vi "test 9401 DIO FPGA Mode Loop Back.vi"(8 "error in (no error)":errorcluster, 11 "TestCase in":refnum<class "Scan Engine EtherCAT System Tests.lvclass">) -> (0 "error out":errorcluster, 3 "TestCase out":refnum<class "Scan Engine EtherCAT System Tests.lvclass">)   [LabVIEW 2019, in "Scan Engine EtherCAT System Tests.lvclass"]
uses:
  Scan Engine EtherCAT System Tests.lvclass
  C:/Users/nitest/Desktop/Git 2019/niveristand-custom-device-testing-tools/VeriStandTestCase/VeriStandTestCase.lvclass
  <vilib>/addons/_JKI Toolkits/VI Tester/TestCase.llb/TestCase.lvclass
  niveristand-custom-device-testing-tools/VeriStandTestCase/VeriStandTestCase.lvclass
  C:/Program Files (x86)/National Instruments/LabVIEW 2019/vi.lib/addons/_JKI Toolkits/VI Tester/TestCase.llb/TestCase.lvclass
  Scan Engine Custom Device.lvlib
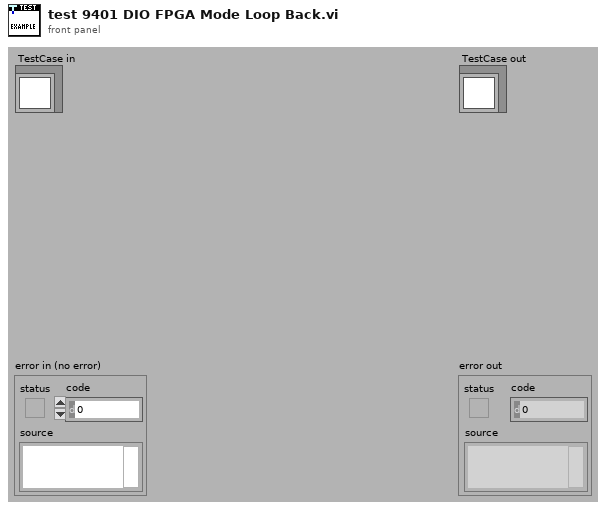
[diagram p1: front panel]
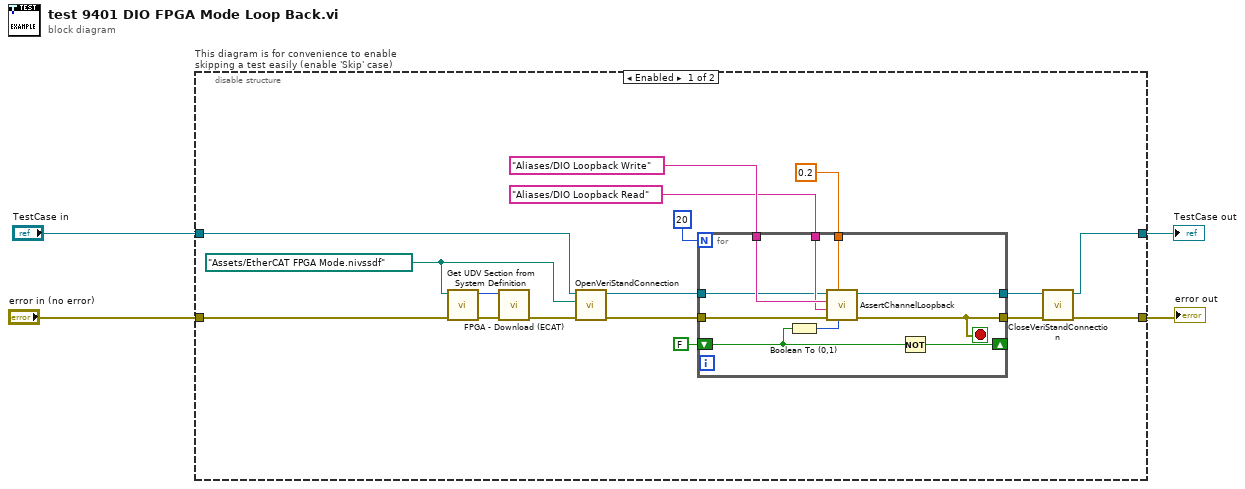
[diagram p0: block diagram]
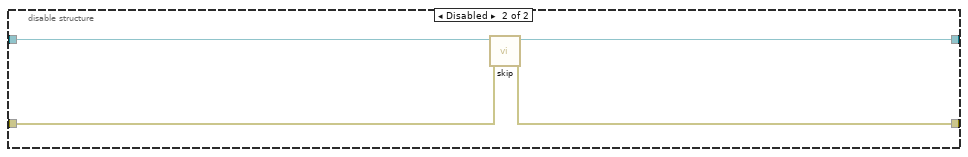
[diagram p2: hidden frame]
diagram:
  n1 = disable-structure "This diagram is for convenience to enable skipping a test easily (enable 'Skip' case)" shown="Enabled" {
    disable-tunnel: "TestCase in" -> [w12 w35]
    disable-tunnel: [w11 w33] -> w1
    disable-tunnel: [w13 w34] -> w3
    disable-tunnel: "error in (no error)" -> [w9 w32]
    frame Enabled {
      w6 = path "Assets/EtherCAT FPGA Mode.nivssdf" ("System Definition File")
      n2 = call "Get UDV Section from System Definition.vi"("error in (no error)"=w9, "System Definition Path"=w6) -> ("error out"=w8:errorcluster, "NodeID"=w5:u64)  [unwired: 8 in]
      n3 = call "FPGA - Download (ECAT).vi"("error in (no error)"=w8, "Node Ptr"=w5) -> ("error out"=w7:errorcluster)  [unwired: 9 in]
      n4 = call-dynamic "OpenVeriStandConnection.vi"("error in (no error)"=w7, "System Definition File"=w6, "VeriStand Test Case in"=w12) -> ("error out"=w17:errorcluster, "VeriStand Test Case out"=w16:refnum<class "Scan Engine EtherCAT System Tests.lvclass">)  [unwired: 6 in, 1 out]
      n5 = for {
        N: 20 -> [_]
        tunnel: "Aliases/DIO Loopback Write" ("Channel") -> [w28]
        tunnel: [w26] -> w15
        tunnel: "Aliases/DIO Loopback Read" ("Channel") -> [w27]
        shift-right: [w31] -> _
        shift-left: FALSE -> [w30]
        tunnel: w17 -> [w29]
        tunnel: [w23] -> w14
        tunnel: w16 -> [w24]
        tunnel: 0.2 ("Delay Time (s)") -> [w22]
        stop <- w26 stop-if-true
        n6 = Boolean To (0,1)(Boolean=w30) -> (0, 1=w25:i16)
        n7 = call "AssertChannelLoopback.vi"("Value"=w25, "Delay Time (s)"=w22, "error in (no error)"=w29, "Read Channel"=w27, "Write Channel"=w28, "VeriStand Test Case in"=w24) -> ("error out"=w26:errorcluster, "VeriStand Test Case out"=w23:refnum<class "Scan Engine EtherCAT System Tests.lvclass">)  [unwired: 4 in]
        n8 = Not(x=w30) -> (.not. x?=w31:bool)
      }
      n9 = call-dynamic "CloseVeriStandConnection.vi"("error in (no error)"=w15, "VeriStand Test Case in"=w14) -> ("error out"=w13:errorcluster, "VeriStand Test Case out"=w11:refnum<class "Scan Engine EtherCAT System Tests.lvclass">)  [unwired: 8 in]
    }
    frame Disabled {
      n10 = call <vilib>:"skip.vi"("error in (no error)"=w32, "TestCase in"=w35) -> ("error out"=w34:errorcluster, "TestCase out"=w33:refnum<class "Scan Engine EtherCAT System Tests.lvclass">)  [unwired: 8 in]
    }
  }
  "error out" <- w3
  "TestCase out" <- w1
